vi "Keyence.Error.vi"(8 "error in (no error)":errorcluster, 9 "Response":string, 10 "Cmd ok":bool=TRUE) -> (0 "error out":errorcluster)   [LabVIEW 2015]
doc: "Desoutter controller error handler\n\n(c) 2013 Test & Measurement Solutions. ALL RIGHTS RESERVED\n\nDeveloped by: Test & Measurement Solutions (www.tm-solutions.pl)\nAuthor: Maciej Szupienko (maciej@tm-solutions.pl)\nReleased at: 05th July 2013"
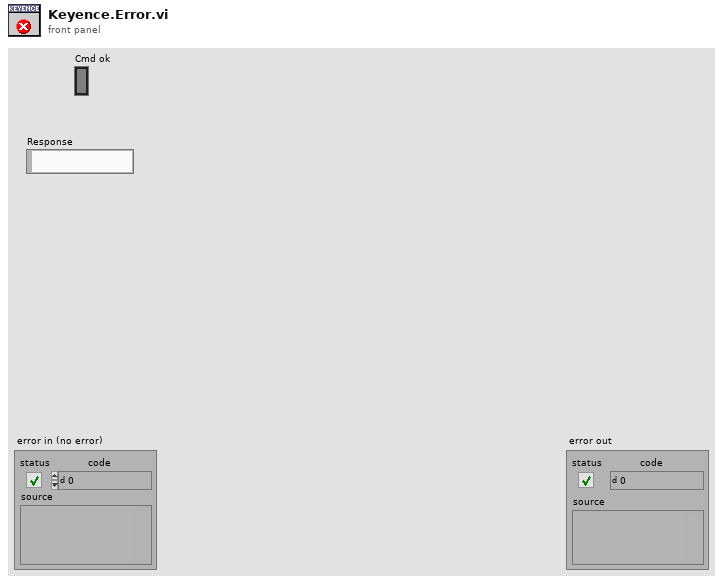
[diagram p1: front panel]
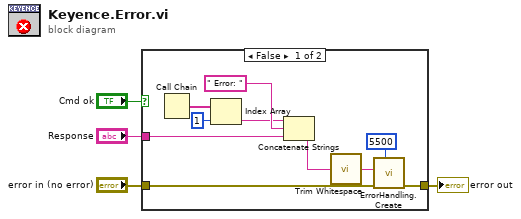
[diagram p0: block diagram]
diagram:
  n1 = case shown="False" "Cmd ok" {
    tunnel: "error in (no error)" -> [w14 w15]
    tunnel: [w13 w15] -> w3
    tunnel: "Response" -> [w7 _]
    frame False {
      n2 = Call Chain() -> (call chain=w12:string[])
      n3 = Index Array(array=w12, index=1) -> (element=w9:string)
      n4 = Concatenate Strings(w9, " Error: " ("format string"), w7) -> (w8:string)
      n5 = call <vilib>:"Trim Whitespace.vi"("string"=w8) -> ("trimmed string"=w5:string)  [unwired: 1 in]
      n6 = call "ErrorHandling.Create.vi"("error code (5000)"=5500 ("error code (0)"), "error in"=w14, "explanation"=w5) -> ("error out"=w13:errorcluster)  [unwired: 8 in]
    }
    frame True {
    }
  }
  "error out" <- w3
